vi "test json to variant cluster.vi"(8 "error in (no error)":errorcluster) -> (0 "error out":errorcluster)   [LabVIEW 2019, in "labview_json_tests.lvlib"]
uses:
  labview_json_tests.lvlib
  lib/labview_json.lvlib
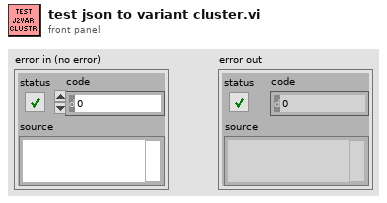
[diagram p1: front panel]
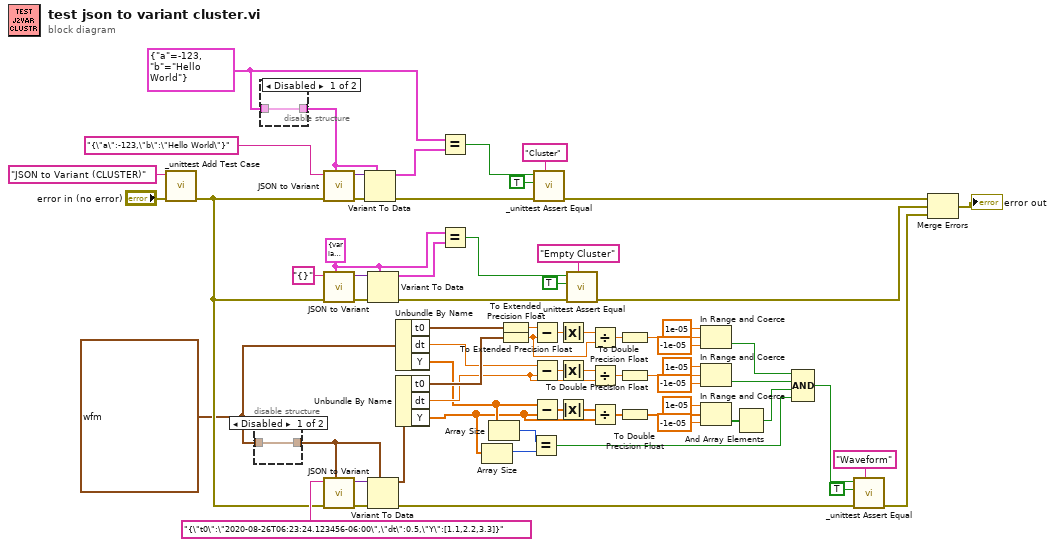
[diagram p0: block diagram]
diagram:
  w43 = waveform(dbl) {"t0"=timestamp(3681289404.123456 s since 1904-01-01), "dt"=0.5, "Y"=[1.1, 2.2, 3.3]} ("Waveform")
  w8 = cluster{variant} {variant} ("Cluster")
  w3 = cluster{"a":i32, "b":string} {"a"=-123, "b"="Hello World"} ("Cluster")
  n1 = call "_unittest Add Test Case.vi"("error in (no error)"="error in (no error)", "Test Case"="JSON to Variant (CLUSTER)") -> ("error out"=w48:errorcluster)  [unwired: 9 in]
  n2 = disable-structure shown="Disabled" {
    disable-tunnel: [w70 _] -> w42
    disable-tunnel: w43 -> [w70 _]
    frame Disabled {
    }
    frame Enabled {
    }
  }
  n3 = disable-structure shown="Disabled" {
    disable-tunnel: [w71 _] -> w56
    disable-tunnel: w3 -> [w71 _]
    frame Disabled {
    }
    frame Enabled {
    }
  }
  n4 = call "JSON to Variant.vi"("Variant Type"=w56, "error in (no error)"=w48, "JSON"="{\"a\":-123,\"b\":\"Hello World\"}") -> ("error out"=w54:errorcluster, "Variant out"=w55:variant)  [unwired: 7 in]
  n5 = call "JSON to Variant.vi"("Variant Type"=w8, "error in (no error)"=w48, "JSON"="{}") -> ("error out"=w65:errorcluster, "Variant out"=w61:variant)  [unwired: 7 in]
  n6 = call "JSON to Variant.vi"("Variant Type"=w42, "error in (no error)"=w48, "JSON"="{\"t0\":\"2020-08-26T06:23:24.123456-06:00\",\"dt\":0.5,\"Y\":[1.1,2.2,3.3]}") -> ("error out"=w49:errorcluster, "Variant out"=w51:variant)  [unwired: 7 in]
  n7 = Variant To Data(error in=w54, type=w56, Variant=w55) -> (data=w4:cluster{"a":i32, "b":string}, error out=w63:errorcluster)
  n8 = Variant To Data(error in=w65, type=w8, Variant=w61) -> (data=w7:cluster{variant}, error out=w62:errorcluster)
  n9 = Variant To Data(error in=w49, type=w42, Variant=w51) -> (data=w46:waveform(dbl), error out=w50:errorcluster)
  n10 = Unbundle By Name(w43) -> ("t0"=w45:timestamp, "dt"=w27:dbl, "Y"=w16:dbl[])
  n11 = Unbundle By Name(w46) -> ("t0"=w44:timestamp, "dt"=w24:dbl, "Y"=w15:dbl[])
  n12 = Equal?(x=w3, y=w4) -> (x = y?=w2:bool)
  n13 = Equal?(x=w8, y=w7) -> (x = y?=w6:bool)
  n14 = Array Size(array=w15) -> (size(s)=w13:i32)
  n15 = Array Size(array=w16) -> (size(s)=w14:i32)
  n16 = To Extended Precision Float(1:w45) -> (0:w40:ext)
  n17 = To Extended Precision Float(1:w44) -> (0:w39:ext)
  n18 = Equal?(x=w14, y=w13) -> (x = y?=w11:bool)
  n19 = Subtract(x=w40, y=w39) -> (x-y=w41:ext)
  n20 = Subtract(x=w27, y=w24) -> (x-y=w28:dbl)
  n21 = Subtract(x=w16, y=w15) -> (x-y=w23:dbl[])
  n22 = call "_unittest Assert Equal.vi"("Message"="Cluster", "error in (no error)"=w63, "Expected Value"=TRUE, "Actual Value"=w2) -> ("error out"=w67:errorcluster)  [unwired: 7 in]
  n23 = Absolute Value(x=w41) -> (abs(x)=w38:ext)
  n24 = Absolute Value(x=w28) -> (abs(x)=w29:dbl)
  n25 = Absolute Value(x=w23) -> (abs(x)=w22:dbl[])
  n26 = call "_unittest Assert Equal.vi"("Message"="Empty Cluster", "error in (no error)"=w62, "Expected Value"=TRUE, "Actual Value"=w6) -> ("error out"=w64:errorcluster)  [unwired: 7 in]
  n27 = Divide(x=w38, y=w39) -> (x/y=w37:ext)
  n28 = Divide(x=w29, y=w24) -> (x/y=w30:dbl)
  n29 = Divide(x=w22, y=w15) -> (x/y=w21:dbl[])
  n30 = To Double Precision Float(number=w37) -> (double precision float=w34:dbl)
  n31 = To Double Precision Float(number=w30) -> (double precision float=w33:dbl)
  n32 = To Double Precision Float(number=w21) -> (double precision float=w18:dbl[])
  n33 = In Range and Coerce(upper limit=1e-05, x=w34, lower limit=-1e-05) -> (In Range?=w26:bool)  [unwired: 1 out]
  n34 = In Range and Coerce(upper limit=1e-05, x=w33, lower limit=-1e-05) -> (In Range?=w25:bool)  [unwired: 1 out]
  n35 = In Range and Coerce(upper limit=1e-05, x=w18, lower limit=-1e-05) -> (In Range?=w17:bool[])  [unwired: 1 out]
  n36 = And Array Elements(Boolean array=w17) -> (logical AND=w12:bool)
  n37 = Compound Arithmetic op=AND(w26, w25, w12, w11) -> (w10:bool)
  n38 = call "_unittest Assert Equal.vi"("Message"="Waveform", "error in (no error)"=w50, "Expected Value"=TRUE, "Actual Value"=w10) -> ("error out"=w47:errorcluster)  [unwired: 7 in]
  n39 = Merge Errors(w67, w64, w47) -> (→"error out":errorcluster)
